vi "settings_load_default_file.vi"(0 "error out":errorcluster) -> ()   [LabVIEW 2010]
uses:
  red_tweezers_globals_INTERNAL_VOLATILE.vi
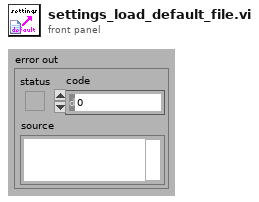
[diagram p1: front panel]
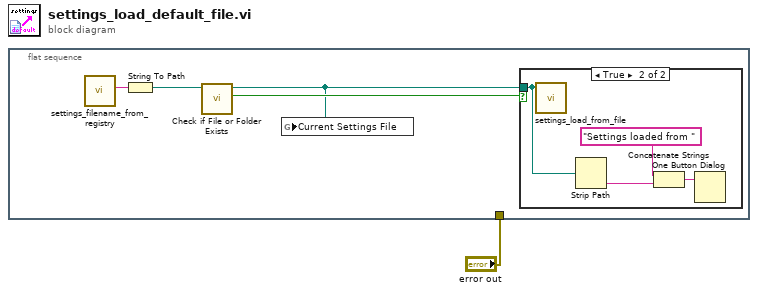
[diagram p0: block diagram]
diagram:
  n1 = flat-sequence {
    tunnel: "error out" -> [_]
    frame #0 {
      n2 = call "settings_filename_from_registry.vi"() -> ("Last Used Settings File"=w5:string)  [unwired: 11 in]
      n3 = String To Path(string=w5) -> (path=w4:path)
      n4 = call <vilib>:"Check if File or Folder Exists.vi"("path"=w4) -> ("file or folder exists?"=w3:bool, "dup path"=w2:path)  [unwired: 8 in, 1 out]
      n5 = global write "red_tweezers_globals_INTERNAL_VOLATILE.vi" "Current Settings File"(w2) -> ()
      n6 = case shown="True" w3 {
        tunnel: w2 -> [_ w6]
        frame False {
        }
        frame True {
          n7 = call "settings_load_from_file.vi"("XML File Path"=w6) -> ()  [unwired: 9 in, 2 out]
          n8 = Strip Path(path=w6) -> (name=w9:string)  [unwired: 1 out]
          n9 = Concatenate Strings("Settings loaded from " ("name"), w9) -> (w7:string)
          n10 = One Button Dialog(message=w7) -> ()  [unwired: 1 in, 1 out]
        }
      }
    }
  }
